vi "Get ID.vi"(11 "Team in":refnum<class "Team.lvclass">) -> (2 "Team ID":T1 format="%.0x")   [LabVIEW 2020, in "SquareBattle.lvlib" / "Team.lvclass"]
doc: "The Team ID is a magic cookie type value that tracks the Game a team was created for and the specific team instance. This value is intended for GUIs and applications that configure game instances and need to track teams uniquely even when their index/ordering changes. This does not provide any value while a game is being run; once a game is started the team index will not change."
uses:
  Team.lvclass
  Team ID.ctl
  Team.lvclass/Team.ctl
  SquareBattle.lvlib
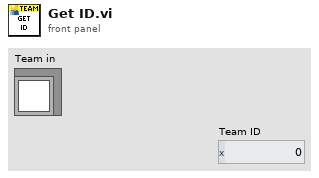
[diagram p1: front panel]
types:
  T1 = typedef "SquareBattle.lvlib/Team ID.ctl" = u32
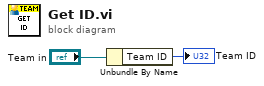
[diagram p0: block diagram]
diagram:
  n1 = Unbundle By Name("Team in") -> ("Team ID"=→"Team ID":T1)
